vi "读取奶茶目录类.vi"(8 "error in (no error)":errorcluster caption="错误输入（无错误）", 11 "奶茶输入":refnum<class "奶茶.lvclass">) -> (0 "error out":errorcluster caption="错误输出", 2 "奶茶目录类":refnum<class>[](array[class]), 3 "奶茶输出":refnum<class "奶茶.lvclass">)   [LabVIEW 2016, in "奶茶.lvclass"]
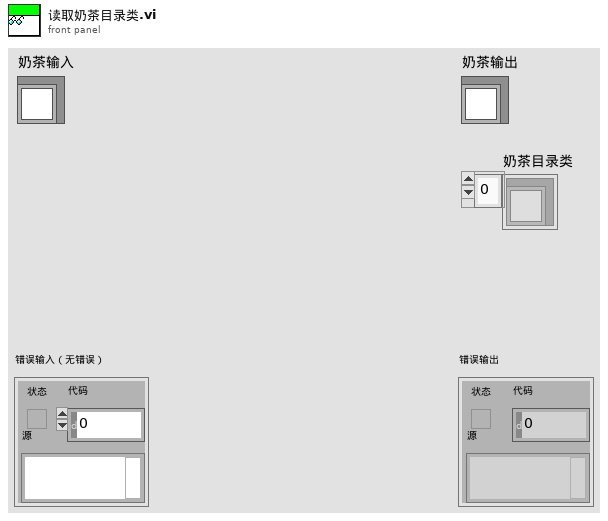
[diagram p1: front panel]
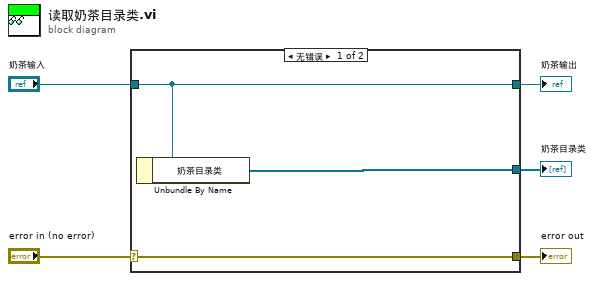
[diagram p0: block diagram]
diagram:
  n1 = case shown="无错误" "error in (no error)" {
    selector: "error in (no error)" -> [w8 w9]
    tunnel: [w8 w9] -> w4
    tunnel: [w7 w10] -> w2
    tunnel: "奶茶输入" -> [w7 w10]
    tunnel: [w6 _] -> w1
    frame No Error {
      n2 = Unbundle By Name(w7) -> ("奶茶目录类"=w6:refnum<class>[])
    }
    frame Error {
    }
  }
  "error out" <- w4
  "奶茶输出" <- w2
  "奶茶目录类" <- w1
